vi "Clean Up Message Queues.vi"(8 "error in (no error)":errorcluster, 11 "Message Queues":T1) -> (0 "error out":errorcluster)   [LabVIEW 2023, in "Weather Message Queue.lvlib"]
doc: "Stops and release all message loops."
uses:
  support/Message Queue/Weather Message Queue.lvlib
  support/Message Queue/All Message Queues.ctl
  support/Message Queue/Message Cluster.ctl
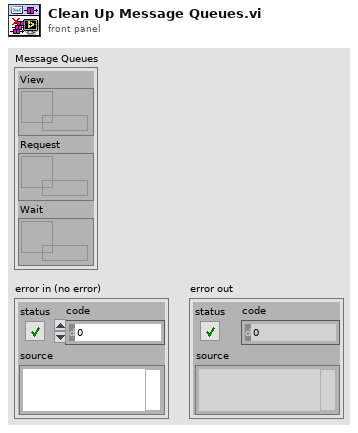
[diagram p1: front panel]
types:
  T1 = typedef "Weather Message Queue.lvlib/All Message Queues.ctl" = cluster{"View":refnum<queue>, "Request":refnum<queue>, "Wait":refnum<queue>}
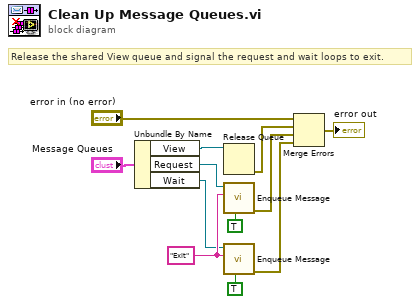
[diagram p0: block diagram]
diagram:
  w7 = "Exit" ("Message")
  # "Release the shared View queue and signal the request and wait loops to exit."
  n1 = Unbundle By Name("Message Queues") -> ("View"=w8:refnum<queue>, "Request"=w6:refnum<queue>, "Wait"=w5:refnum<queue>)
  n2 = Release Queue(queue=w8) -> (error out=w12:errorcluster)  [unwired: 2 in, 2 out]
  n3 = call "Enqueue Message.vi"("Priority Message? (F)"=TRUE, "Message"=w7, "Message Queue"=w6) -> ("error out"=w11:errorcluster)  [unwired: 7 in, 1 out]
  n4 = call "Enqueue Message.vi"("Priority Message? (F)"=TRUE, "Message"=w7, "Message Queue"=w5) -> ("error out"=w10:errorcluster)  [unwired: 7 in, 1 out]
  n5 = Merge Errors("error in (no error)", w12, w11, w10) -> (→"error out":errorcluster)
